vi "Path.vi"() -> (0 "error out":errorcluster, 3 "Path":path)   [LabVIEW 2021, in "File Library.lvlib" / "User Connections.lvclass"]
uses:
  User Connections.lvclass
  <vilib>/Utility/sysdir.llb/System Directory Type.ctl
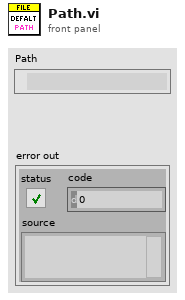
[diagram p1: front panel]
types:
  T1 = typedef "System Directory Type.ctl" = i32
  T2 = enum16{"open", "replace", "create", "open or create", "replace or create", "replace or create with confirmation"}
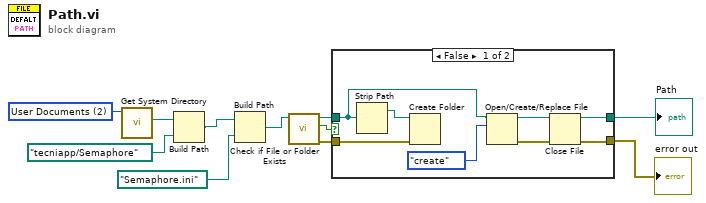
[diagram p0: block diagram]
diagram:
  w11 = T1 2 items=["User Home"=0, "User Desktop"=1, "User Documents"=2, "User Application Data"=3, "User Preferences"=4, "User Temporary"=5, "Public Documents"=6, "Public Application Data"=7, "Public Preferences"=8, "Public Cache"=13, "System Core Libraries"=9, "System Installed Libraries"=10, "Application Files"=11, "Boot Volume Root"=12] ("system directory type")
  n1 = call <vilib>:"Get System Directory.vi"("system directory type"=w11) -> ("system directory"=w10:path)  [unwired: 10 in]
  n2 = Build Path(base path=w10, name or relative path=path "tecniapp/Semaphore") -> (appended path=w3:path)
  n3 = Build Path(base path=w3, name or relative path=path "Semaphore.ini") -> (appended path=w2:path)
  n4 = call <vilib>:"Check if File or Folder Exists.vi"("path"=w2) -> ("error out"=w7:errorcluster, "file or folder exists?"=w4:bool, "dup path"=w8:path)  [unwired: 8 in]
  n5 = case shown="False" w4 {
    tunnel: w8 -> [w13 w21]
    tunnel: w7 -> [w19 w20]
    tunnel: [w15 w20] -> w6
    tunnel: [w14 w21] -> w5
    frame False {
      n6 = Strip Path(path=w13) -> (stripped path=w18:path)  [unwired: 1 out]
      n7 = Create Folder(path (use dialog)=w18, error in=w19) -> ()  [unwired: 1 in, 3 out]
      n8 = Open/Create/Replace File(file path (use dialog)=w13, operation (0:open)=T2."create") -> (refnum out=w17:refnum<file>, error out=w16:errorcluster)  [unwired: 4 in, 1 out]
      n9 = Close File(refnum=w17, error in=w16) -> (path=w14:path, error out=w15:errorcluster)
    }
    frame True {
    }
  }
  "Path" <- w5
  "error out" <- w6
